vi "priklad.vi"() -> ()   [LabVIEW 2013]
uses:
  Private/Add key polymorph parts/EXT.vi
  Private/Add key polymorph parts/String.vi
  Private/Add matrix polymorph parts/2D EXT.vi
  Private/Add key polymorph parts/Time Stamp.vi
  infolib.lvlib
panel:
  out "info data out":string
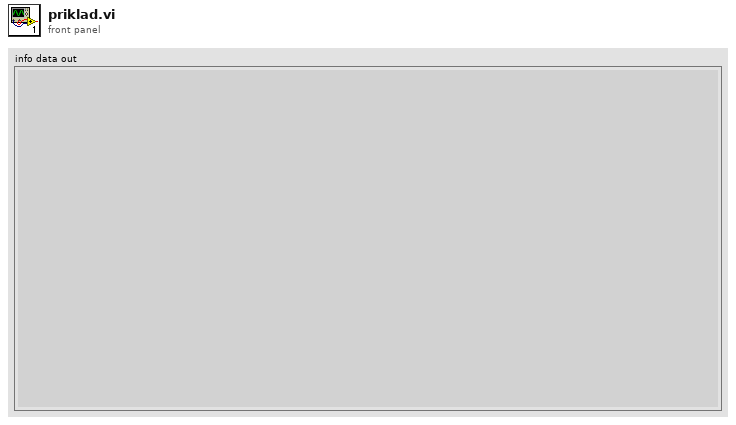
[diagram p1: front panel]
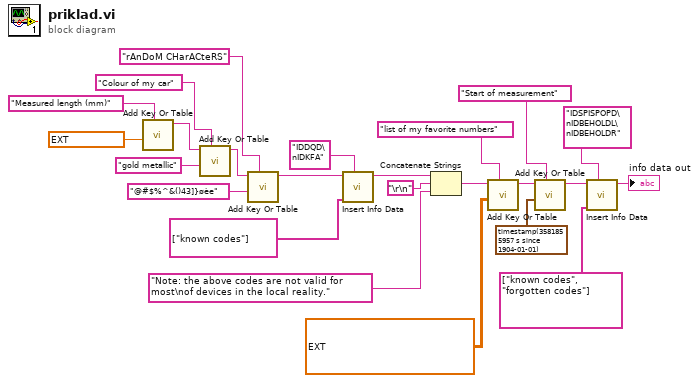
[diagram p0: block diagram]
diagram:
  n1 = call-poly "Add Key Or Table.vi"("key description"="Measured length (mm)", "numeric"=ext 34.123456789) -> ("info data out"=w22:string)  [unwired: 8 in, 1 out]
  n2 = call-poly "Add Key Or Table.vi"("key description"="Colour of my car", "string"="gold metallic" ("key description"), "info data"=w22) -> ("info data out"=w17:string)  [unwired: 7 in, 1 out]
  n3 = call-poly "Add Key Or Table.vi"("key description"="rAnDoM CHarACteRS", "string"="@#$%^&()43]}øèe" ("key description"), "info data"=w17) -> ("info data out"=w16:string)  [unwired: 7 in, 1 out]
  n4 = call "Insert Info Data.vi"("info data to insert"="IDDQD\nIDKFA" ("key description"), "sections"=string[] ["known codes"], "info data"=w16) -> ("info data out"=w13:string)  [unwired: 7 in, 1 out]
  n5 = Concatenate Strings(w13, "\r\n", "Note: the above codes are not valid for most\nof devices in the local reality." ("string")) -> (w10:string)
  n6 = call-poly "Add Key Or Table.vi"("key description"="list of my favorite numbers", "numeric"=ext[][] [[1.0, 11.0, 42.0], [3333.0, 1e+72, 0.0], [-1.0, -3333.0, 0.00000100000000000000000004]], "info data"=w10) -> ("info data out"=w7:string)  [unwired: 7 in, 1 out]
  n7 = call-poly "Add Key Or Table.vi"("key description"="Start of measurement", "time stamp"=timestamp(3581855957.019788 s since 1904-01-01), "info data"=w7) -> ("info data out"=w6:string)  [unwired: 7 in, 1 out]
  n8 = call "Insert Info Data.vi"("info data to insert"="IDSPISPOPD\nIDBEHOLDL\nIDBEHOLDR", "sections"=string[] ["known codes", "forgotten codes"], "info data"=w6) -> ("info data out"=→"info data out":string)  [unwired: 7 in, 1 out]
